vi "Global 1.vi"() -> ()   [LabVIEW 2023]
panel:
  out "Boolean":bool
  out "new file path (Not A Path if cancelled)":path
  in  "task out":refnum<k21>
  in  "error out":errorcluster
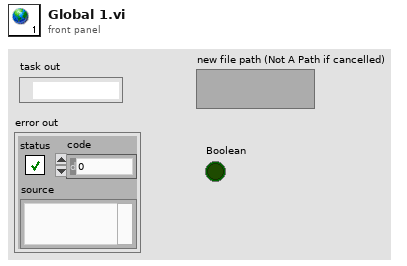
[diagram p1: front panel]
diagram:
